vi "Read.vi"(8 "error in (no error)":errorcluster, 11 "Double Float.lvclass in":refnum<class "Subtract_Time.lvclass">) -> (0 "error out":errorcluster, 2 "Value":timestamp, 3 "Double Float.lvclass out":refnum<class "Subtract_Time.lvclass">)   [LabVIEW 2021, in "Subtract_Time.lvclass"]
uses:
  Subtract_Time.lvclass
  Subtract_Time.lvclass/Subtract_Time.ctl
  Abs_Types/Time/Abs_Time.lvclass
  Abs_Types/Numeric/Abs_Numeric.lvclass
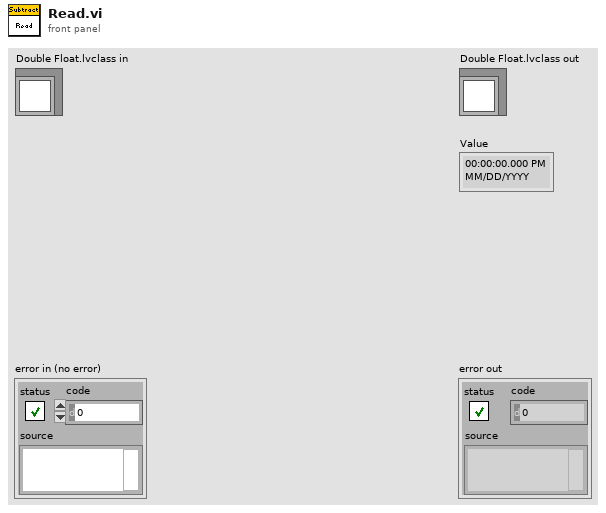
[diagram p1: front panel]
types:
  T1 = typedef "Abs_Time.lvclass/Type.ctl" = timestamp
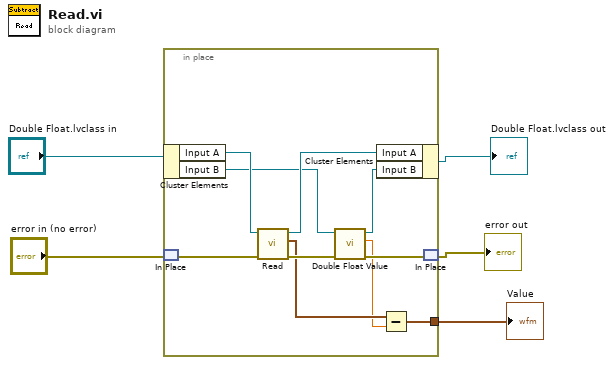
[diagram p0: block diagram]
diagram:
  n1 = in-place {
    in-place-border: [w6] -> w1
    n2 = in-place-cluster #1("Double Float.lvclass in") -> ("Input A"=w15:refnum<class "Abs_Time.lvclass">, "Input B"=w13:refnum<class "Abs_Numeric.lvclass">)
    n3 = in-place-match #2("error in (no error)") -> (w11:errorcluster)
    n4 = call-dynamic "Read.vi"("error in (no error)"=w11, "Double Float.lvclass_340760 in"=w15) -> ("error out"=w10:errorcluster, "Value"=w8:T1, "Double Float.lvclass_340760 out"=w14:refnum<class "Abs_Time.lvclass">)  [unwired: 7 in]
    n5 = call-dynamic "Double Float Value.vi"("error in (no error)"=w10, "Numeric in"=w13) -> ("error out"=w9:errorcluster, "Double"=w7:dbl, "Numeric out"=w12:refnum<class "Abs_Numeric.lvclass">)  [unwired: 7 in]
    n6 = in-place-cluster #1("Input A"=w14, "Input B"=w12) -> (→"Double Float.lvclass out":refnum<class "Subtract_Time.lvclass">)
    n7 = Subtract(x=w8, y=w7) -> (x-y=w6:T1)
    n8 = in-place-match #2(w9) -> (→"error out":errorcluster)
  }
  "Value" <- w1
